vi "Setfocus - manual.vi"(9 "#steps":i32=100, 10 "Z end (V)":dbl=10.0 format="%.2f", 11 "Z start (V)":dbl) -> ()   [LabVIEW 2014]
uses:
  global_variables_AWG.vi
  global_channels.vi
panel:
  in  "Focus smoothing":bool
  in  "Offset":bool
  out "counts 2":u32=19340
  out "Waveform Chart":dbl(graph)=19340.0
  in  "Get Counts":bool
  in  "acquisition time per point (s)":dbl=0.1 format="%.3f"
  out "Z position out":dbl
  in  "Cancel":bool
  out "duration (s)":dbl=10.0 format="%#_6p"
  in  "Done":bool
  in  "Start Scan":bool
  out "Z-position":dbl
  out "Y-position":dbl
  out "X-position":dbl
  out "Z cursor position":dbl format="%.3g"
  in  "time per point (s)":dbl=0.1 format="%#_6p"
  out "Z focus":cluster{dbl[], "histogram plot":dbl[]}(graph)={[0.0, 0.1, 0.2, 0.30000000000000004, 0.4, 0.5, 0.6, 0.7, 0.7999999999999999, 0.8999999999999999, 0.9999999999999999, 1.0999999999999999, 1.2, 1.3, 1.4000000000000001, 1.5000000000000002, 1.6000000000000003, 1.7000000000000004, 1.8000000000000005, 1.9000000000000006, 2.0000000000000004, 2.1000000000000005, 2.2000000000000006, 2.3000000000000007, 2.400000000000001, 2.500000000000001, 2.600000000000001, 2.700000000000001, 2.800000000000001, 2.9000000000000012, 3.0000000000000013, 3.1000000000000014, 3.2000000000000015, 3.3000000000000016, 3.4000000000000017, 3.5000000000000018, 3.600000000000002, 3.700000000000002, 3.800000000000002, 3.900000000000002, 4.000000000000002, 4.100000000000001, 4.200000000000001, 4.300000000000001, 4.4, 4.5, 4.6, 4.699999999999999, 4.799999999999999, 4.899999999999999, 4.999999999999998, 5.099999999999998, 5.1999999999999975, 5.299999999999997, 5.399999999999997, 5.4999999999999964, 5.599999999999996, 5.699999999999996, 5.799999999999995, 5.899999999999995, 5.999999999999995, 6.099999999999994, 6.199999999999994, 6.299999999999994, 6.399999999999993, 6.499999999999993, 6.5999999999999925, 6.699999999999992, 6.799999999999992, 6.8999999999999915, 6.999999999999991, 7.099999999999991, 7.19999999999999, 7.29999999999999, 7.39999999999999, 7.499999999999989, 7.599999999999989, 7.699999999999989, 7.799999999999988, 7.899999999999988, 7.999999999999988, 8.099999999999987, 8.199999999999987, 8.299999999999986, 8.399999999999986, 8.499999999999986, 8.599999999999985, 8.699999999999985, 8.799999999999985, 8.899999999999984, 8.999999999999984, 9.099999999999984, 9.199999999999983, 9.299999999999983, 9.399999999999983, 9.499999999999982, 9.599999999999982, 9.699999999999982, 9.799999999999981, 9.89999999999998, 9.99999999999998], "histogram plot"=[200.0, 110.0, 100.0, 130.0, 130.0, 210.0, 150.0, 150.0, 170.0, 130.0, 110.0, 180.0, 210.0, 160.0, 110.0, 180.0, 100.0, 120.0, 200.0, 200.0, 130.0, 70.0, 140.0, 150.0, 120.0, 140.0, 200.0, 110.0, 140.0, 150.0, 150.0, 200.0, 150.0, 150.0, 160.0, 80.0, 140.0, 100.0, 200.0, 170.0, 190.0, 160.0, 200.0, 300.0, 270.0, 230.0, 230.0, 230.0, 230.0, 280.0, 300.0, 110.0, 250.0, 320.0, 180.0, 200.0, 220.0, 330.0, 210.0, 250.0, 210.0, 200.0, 160.0, 180.0, 240.0, 180.0, 240.0, 170.0, 240.0, 170.0, 170.0, 140.0, 140.0, 180.0, 130.0, 210.0, 130.0, 170.0, 100.0, 150.0, 100.0, 170.0, 150.0, 140.0, 210.0, 180.0, 150.0, 140.0, 100.0, 250.0, 150.0, 170.0, 80.0, 140.0, 190.0, 130.0, 130.0, 80.0, 110.0, 100.0, 180.0]}
  # "Automatic => Press \"Start Scan\n\nManual => Move cursor"
  # "Current XYZ"
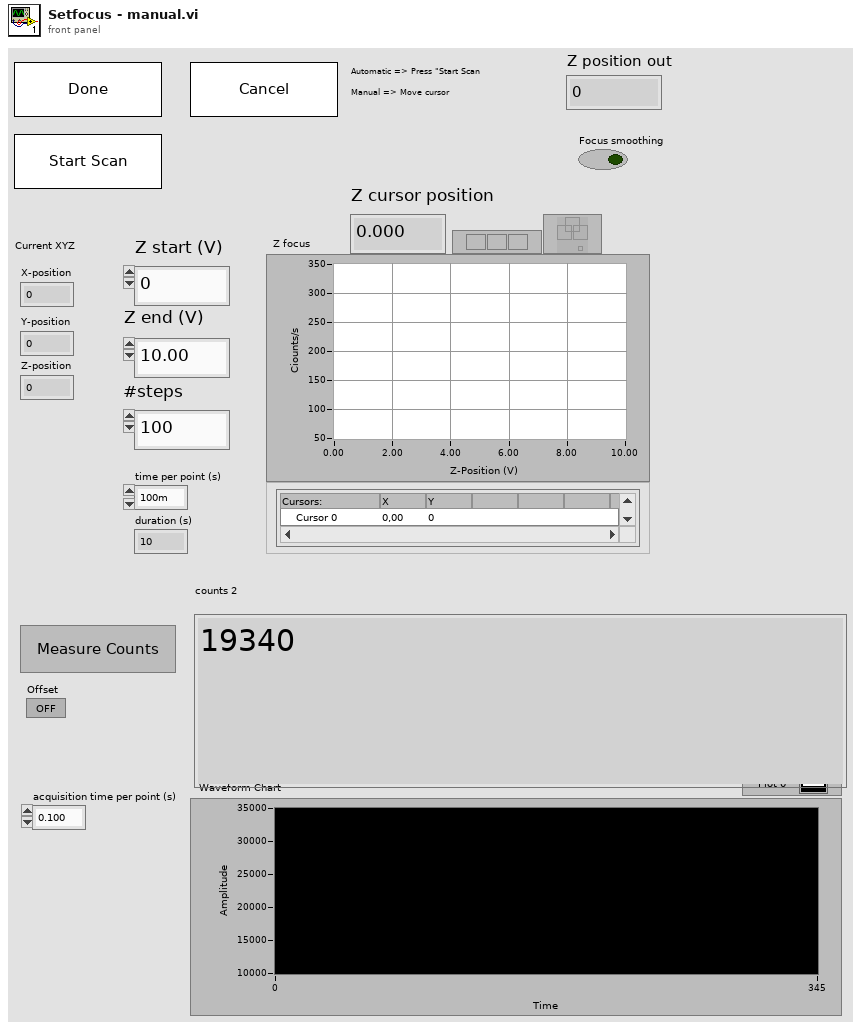
[diagram p1: front panel]
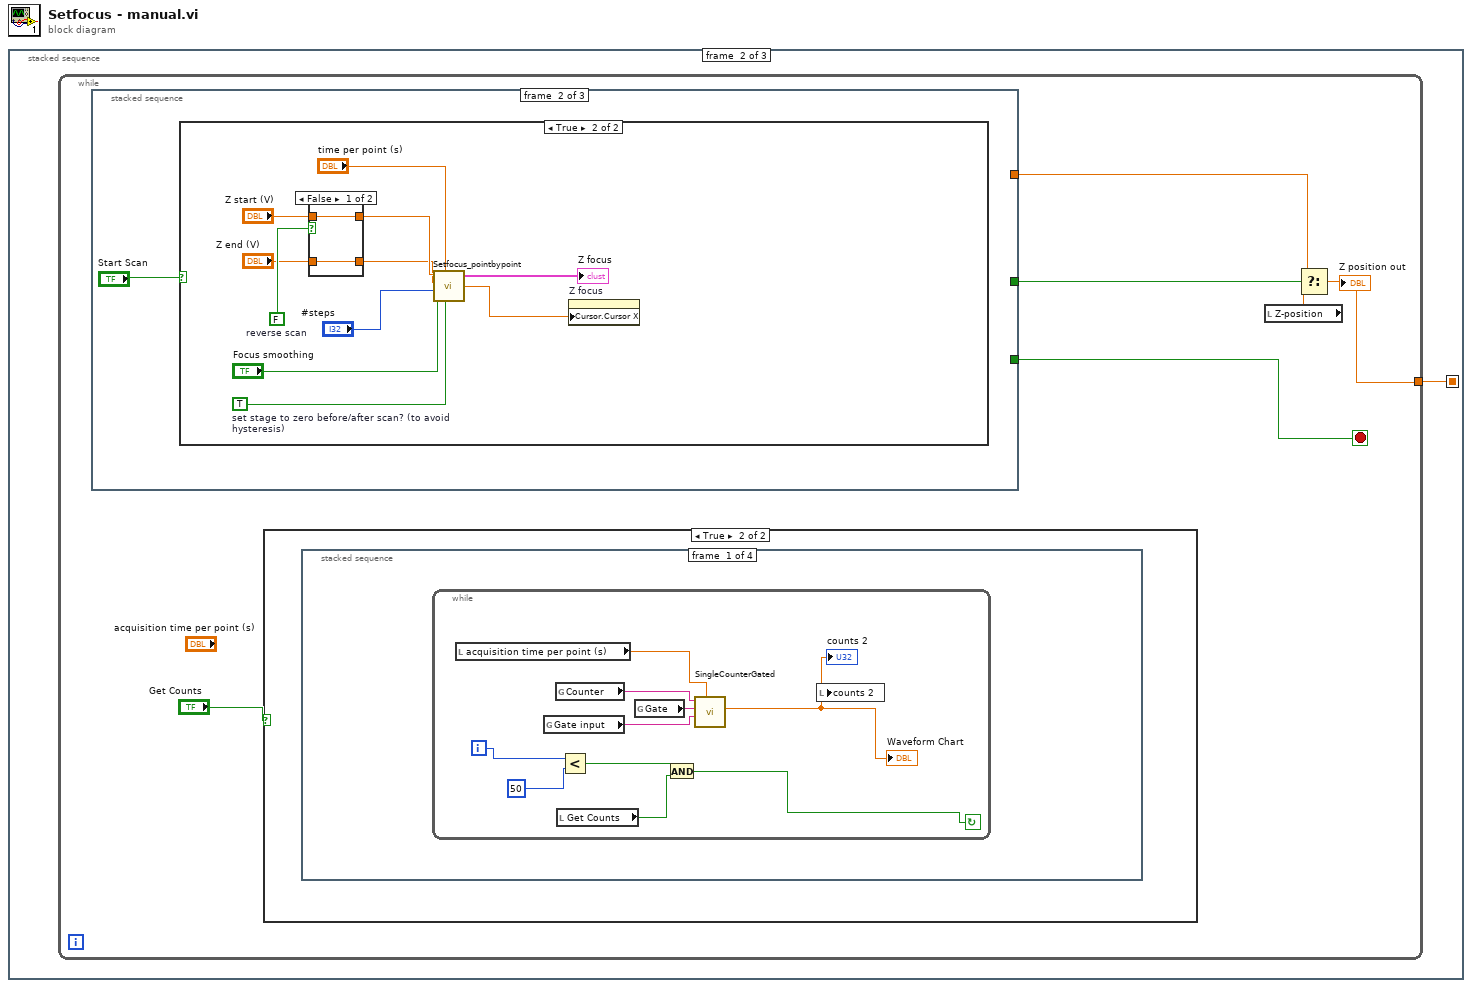
[diagram p0: block diagram]
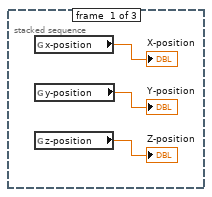
[diagram p2: hidden frame]
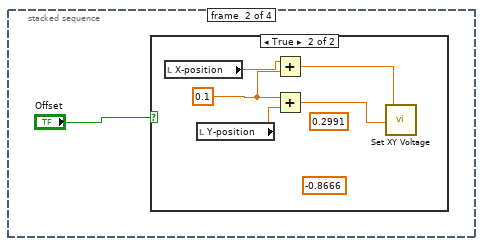
[diagram p4: hidden frame]
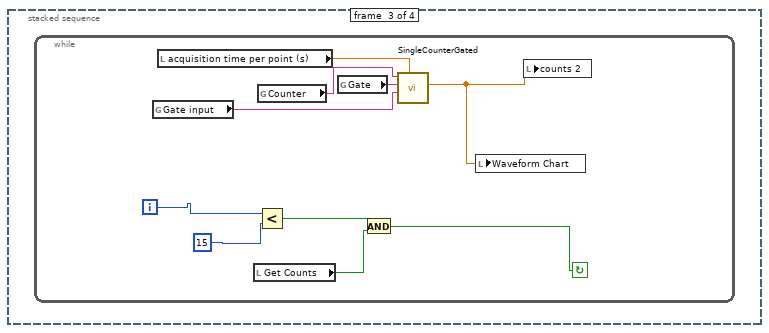
[diagram p6: hidden frame]
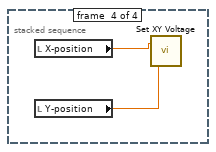
[diagram p7: hidden frame]
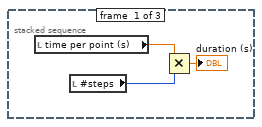
[diagram p8: hidden frame]
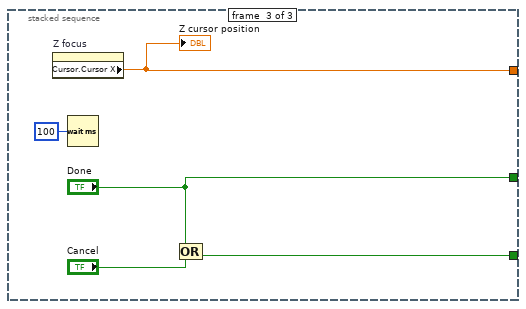
[diagram p11: hidden frame]
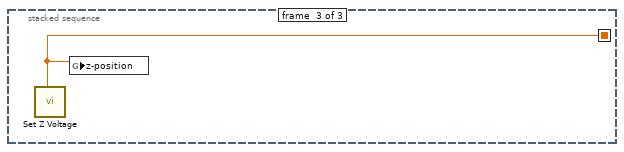
[diagram p12: hidden frame]
diagram:
  n1 = stacked-sequence {
    seq-local: [_ w4 _] -> [_ _ w63]
    frame #0 {
      n2 = global read "global_variables_AWG.vi" "x-position"() -> (→"X-position":dbl)
      n3 = global read "global_variables_AWG.vi" "y-position"() -> (→"Y-position":dbl)
      n4 = global read "global_variables_AWG.vi" "z-position"() -> (→"Z-position":dbl)
    }
    frame #1 {
      n5 = while {
        tunnel: [w6] -> w4
        stop <- w10 stop-if-true
        n6 = stacked-sequence {
          tunnel: [_ _ w61] -> w10
          tunnel: [_ _ "Done"] -> w9
          tunnel: [_ _ w58] -> w7
          frame #0 {
            n7 = local read "time per point (s)"() -> (w41:dbl)
            n8 = local read "#steps"() -> (w40:i32)
            n9 = Multiply(x=w41, y=w40) -> (x*y=→"duration (s)":dbl)
          }
          frame #1 {
            n10 = case shown="True" "Start Scan" {
              frame False {
              }
              frame True {
                w44 = TRUE  # set stage to zero before/after scan? (to avoid hysteresis)
                w53 = FALSE  # reverse scan
                n11 = case shown="False" w53 {
                  tunnel: "Z end (V)" -> [w54 w56]
                  tunnel: "Z start (V)" -> [w55 w57]
                  tunnel: [w55 w56] -> w47
                  tunnel: [w54 w57] -> w46
                  frame False {
                  }
                  frame True {
                  }
                }
                n12 = call "Setfocus_pointbypoint.vi"("Z start (V)"=w47, "time per point (s)"="time per point (s)", "Z end (V)"=w46, "#steps"="#steps", "set stage to zero before scan? (to avoid hysteresis)"=w44, "Focus smoothing"="Focus smoothing") -> ("Z focus 2"=→"Z focus":cluster{dbl[], "histogram plot":dbl[]}, "Z max (V)"=w49:dbl)  [unwired: 1 in]
                n13 = property on="Z focus" class="XYGraph (strict)"("Cursor.Cursor X"=w49) -> ()  [unwired: 2 in, 2 out]
              }
            }
          }
          frame #2 {
            n14 = property on="Z focus" class="XYGraph (strict)"() -> ("Cursor.Cursor X"=w58:dbl)  [unwired: 2 in, 2 out]
            "Z cursor position" <- w58
            n15 = Wait (ms)(milliseconds to wait=u32 100) -> ()  [unwired: 1 out]
            n16 = Compound Arithmetic op=OR("Done", "Cancel") -> (w61:bool)
          }
        }
        n17 = case shown="True" "Get Counts" {
          frame False {
          }
          frame True {
            n18 = stacked-sequence {
              frame #0 {
                n19 = while {
                  i -> [w15]
                  stop <- w11 continue-if-true
                  n20 = local read "acquisition time per point (s)"() -> (w17:dbl)
                  n21 = global read "global_channels.vi" "Gate input"() -> (w18:tag)
                  n22 = global read "global_channels.vi" "Counter"() -> (w20:tag)
                  n23 = local read "Get Counts"() -> (w13:bool)
                  n24 = Less?(x=w15, y=50) -> (x < y?=w12:bool)
                  n25 = global read "global_channels.vi" "Gate"() -> (w19:tag)
                  n26 = And(x=w12, y=w13) -> (x .and. y?=w11:bool)
                  n27 = call "SingleCounterGated.vi"("Acquisition time [s]"=w17, "Gate input"=w18, "Gate"=w19, "Counter"=w20) -> ("counts/s"=w16:dbl)  [unwired: 5 in, 2 out]
                  "counts 2" <- w16
                  "Waveform Chart" <- w16
                  n28 = local write "counts 2"(w16) -> ()
                }
              }
              frame #1 {
                n29 = case shown="True" "Offset" {
                  frame False {
                  }
                  frame True {
                    (unwired) -0.8666
                    (unwired) 0.2991
                    w24 = 0.1 ("X-Position")
                    n30 = local read "X-position"() -> (w25:dbl)
                    n31 = local read "Y-position"() -> (w26:dbl)
                    n32 = Add(x=w25, y=w24) -> (x+y=w23:dbl)
                    n33 = Add(x=w24, y=w26) -> (x+y=w22:dbl)
                    n34 = call "Set XY Voltage.vi"("Y-Position"=w22, "X-Position"=w23) -> ()  [unwired: 1 in]
                  }
                }
              }
              frame #2 {
                n35 = while {
                  i -> [w28]
                  stop <- w29 continue-if-true
                  n36 = global read "global_channels.vi" "Gate input"() -> (w35:tag)
                  n37 = local read "acquisition time per point (s)"() -> (w36:dbl)
                  n38 = local read "Get Counts"() -> (w31:bool)
                  n39 = Less?(x=w28, y=15) -> (x < y?=w30:bool)
                  n40 = global read "global_channels.vi" "Counter"() -> (w33:tag)
                  n41 = global read "global_channels.vi" "Gate"() -> (w34:tag)
                  n42 = And(x=w30, y=w31) -> (x .and. y?=w29:bool)
                  n43 = call "SingleCounterGated.vi"("Acquisition time [s]"=w36, "Gate input"=w35, "Gate"=w34, "Counter"=w33) -> ("counts/s"=w32:dbl)  [unwired: 5 in, 2 out]
                  n44 = local write "Waveform Chart"(w32) -> ()
                  n45 = local write "counts 2"(w32) -> ()
                }
              }
              frame #3 {
                n46 = local read "X-position"() -> (w38:dbl)
                n47 = local read "Y-position"() -> (w37:dbl)
                n48 = call "Set XY Voltage.vi"("Y-Position"=w37, "X-Position"=w38) -> ()  [unwired: 1 in]
              }
            }
          }
        }
        n49 = local read "Z-position"() -> (w8:dbl)
        n50 = Select(t=w7, s=w9, f=w8) -> (s? t:f=w6:dbl)
        "Z position out" <- w6
      }
    }
    frame #2 {
      n51 = call "Set Z Voltage.vi"("Z position (V)"=w63) -> ()  [unwired: 2 in]
      n52 = global write "global_variables_AWG.vi" "z-position"(w63) -> ()
    }
  }
